vi "Configure Active DUT Control User Prompt Timeout.vi"(8 "error in (no error)":errorcluster, 10 "User Prompt Timeout (10)":dbl=10.0 format="%^.3e", 11 "VISA resource name":refnum<visa-resource-name>) -> (0 "error out":errorcluster, 3 "VISA resource name out":refnum<visa-resource-name>)   [LabVIEW 2020, in "Rohde&Schwarz CMXP Base.lvlib"]
doc: "Specifies the no answer timeout for a DUT action in manual control mode.\n\nAttribute:\nRSCMXPBASE_ATTR_ACTIVE_DUT_CONTROL_USER_PROMPT_TIMEOUT\n\nRemote-control command:\n[CONFigure:]DUT:CONTrol:MANual:UPTout"
uses:
  <instrlib>/Rohde&Schwarz CMXP Base/Rohde&Schwarz CMXP Base.lvlib
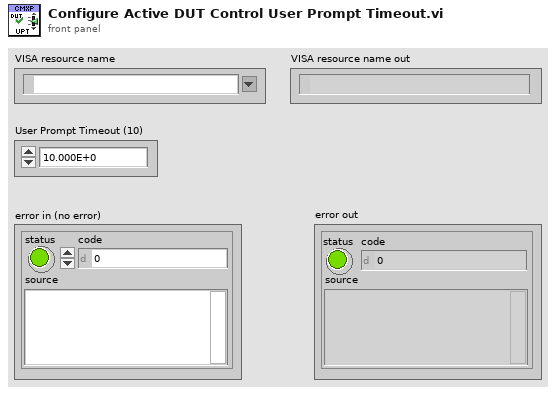
[diagram p1: front panel]
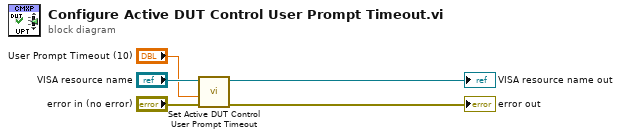
[diagram p0: block diagram]
diagram:
  n1 = call "Set Active DUT Control User Prompt Timeout"("error in (no error)"="error in (no error)", "Active DUT Control User Prompt Timeout (0.0)"="User Prompt Timeout (10)", "instrument handle"="VISA resource name") -> ("error out"=→"error out":errorcluster, "instrument handle out"=→"VISA resource name out":refnum<visa-resource-name>)  [unwired: 7 in]
